vi "trace_data_compute_extra.vi"(0 "Input Trace":sgl[][](array[numeric])) -> (2 "Full Trace":sgl[][](array[numeric]))   [LabVIEW 2014]
uses:
  probe_point.ctl
  pose_source.ctl
  <vilib>/Analysis/baseanly.llb/A x Vector.vi
  initialization/micron_globals.vi
  <vilib>/Analysis/NI_AALBase.lvlib
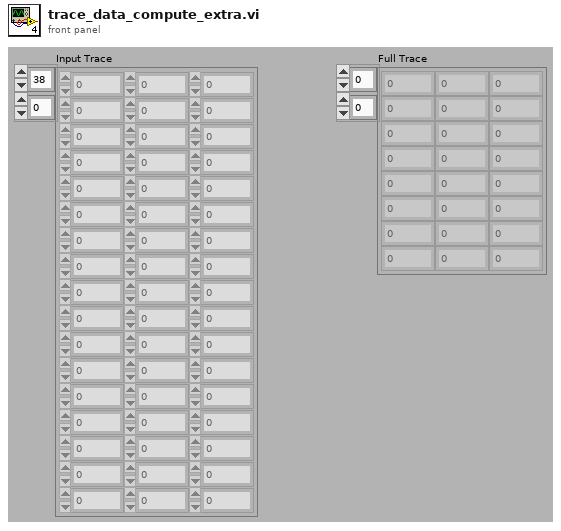
[diagram p1: front panel]
types:
  T1 = typedef "probe_point.ctl" = enum16{"Position (tip)", "Position (RCM)", "Null pos (tip)", "Null pos (RCM)", "V limiter (tip)", "V Limiter (RCM)", "Goal filter (tip)", "Goal filter (RCM)", "Goal force (tip)", "Goal force (RCM)", "Goal (tip)", "Goal (RCM)", "Link pos 0", "Link pos 1", "KF link pos 0", "KF link pos 1", "Link rate 0", "Link rate 1", "Link residue 0", "Link residue 1", "Link goal 0", "Link goal 1", "Rate limit 0", "Rate limit 1", "Link error 0", "Link error 1", "Controller 0", "Controller 1", "Output 0", "Output 1", "Drive 0", "Drive 1", "Stimulus 0", "Stimulus 1", "Trace data 0", "Trace data 1", "Analog data 0", "Analog data 1", "Status flags", "Light 0", "Light 1", "Light 2", "Light 3", "Light 4", "Light 5", "Goal origin", "Goal rotation 0", "Goal rotation 1", "Goal rotation 2", "Output origin", "Output rotation 0", "Output rotation 1", "Output rotation 2", "Handle origin", "Handle rotation 0", "Handle rotation 1", "Handle rotation 2", "Handle position", "Handle velocity", "Handle acceleration", "Handle angles", "Handle angle rates", "Handle pos residue", "Handle angle residue", "Trace length"}
  T2 = typedef "pose_source.ctl" = enum16{"Output", "Handle", "Handle KF", "Goal", "Absolute"}
  T3 = typedef "Micron params.ctl" = cluster{"Stimulus":T4, "Goal Filter A":T6, "Mode controls":T7, "Manipulator type":enum16{"Current piezo", "Voltage piezo"}, "Manipulator calibration":T8, "Network":T10, "Goal Filter B":T6, "Cancellation":T11, "Transition time":sgl, "Estimation":T13}
  T4 = typedef "stimulus.ctl" = cluster{"Type":enum16{"Off", "Step", "Sine", "Triangle", "Arbitrary"}, "Phase":dbl, "Amplitude":sgl[], "Injection point":T5, "Closed loop":bool, "Offset":sgl[], "Tip -> world":bool, "Frequency":dbl, "Length":dbl}
  T5 = typedef "injection_point.ctl" = enum16{"Total pose", "V limiter", "Goal ", "Link position", "KF link position", "Inverse kin", "Link goal", "Link error", "Controller", "Output", "Drive", "Light"}
  T6 = typedef "goal_loop_parms.ctl" = cluster{"Speedup max":sgl, "Speedup thresh":sgl, "Speedup nonlin":sgl, "Filters":cluster{"Lower Fc":sgl, "Lower Q":sgl, "Scale factor":sgl, "Upper Fc":sgl, "Upper Q":sgl, "V limit":sgl, "V limit range":sgl}[]}
  T7 = typedef "mode_conrols.ctl" = cluster{"Hold":bool, "Cancellation":bool, "Goal filter":bool, "Trigger":bool}
  T8 = typedef "manipulator_cal.ctl" = cluster{"Tool offsets":sgl[][], "Tip light calibration":T9, "Handle light calibration":T9, "Base pivots":sgl[][], "Output pivots":sgl[][], "Length center":sgl, "Workspace height":sgl[], "Workspace diameter":sgl[], "Linearization":sgl[][], "Stack travel":sgl, "Saturation pos":sgl, "Inverse filters":cluster{"filter structure":enum32{"IIR 2nd Order", "IIR 4th Order"}, "Reverse Coefficients":dbl[], "Forward Coefficients":dbl[]}[]}
  T9 = typedef "probe_calibration.ctl" = sgl[][]
  T10 = typedef "network_params.ctl" = cluster{"Remote Host":string, "Send Status":bool, "Send Port":u16, "Recv Commands":bool, "Recv Port":u16}
  T11 = typedef "sq_control_params.ctl" = cluster{"KP":T12, "KI":sgl, "KD":T12, "Max vel":sgl, "Max acc":sgl, "Int error limit":sgl, "RCM gain":sgl, "Bypass":bool, "Degraded gain":sgl}
  T12 = typedef "decoupled_gain.ctl" = cluster{"XY":sgl, "Rxy":sgl, "Z":sgl, "Rz":sgl}
  T13 = typedef "estimation_controls.ctl" = cluster{"Link":cluster{"Measure noise":dbl[], "Process noise":dbl[], "Alt process noise":dbl[], "Alt turnoff cycles":i32, "Innovation limit":dbl[], "Residue threshold":dbl, "Enable":bool}, "Handle":cluster{"Measure noise":dbl[], "Process noise":dbl[], "State limits":dbl[], "Innovation limit":dbl[], "Prediction Lookahead":sgl, "Enable":bool}}
  T14 = typedef "NI_Matrix.lvlib/RealMatrix.ctl" = dbl[][]
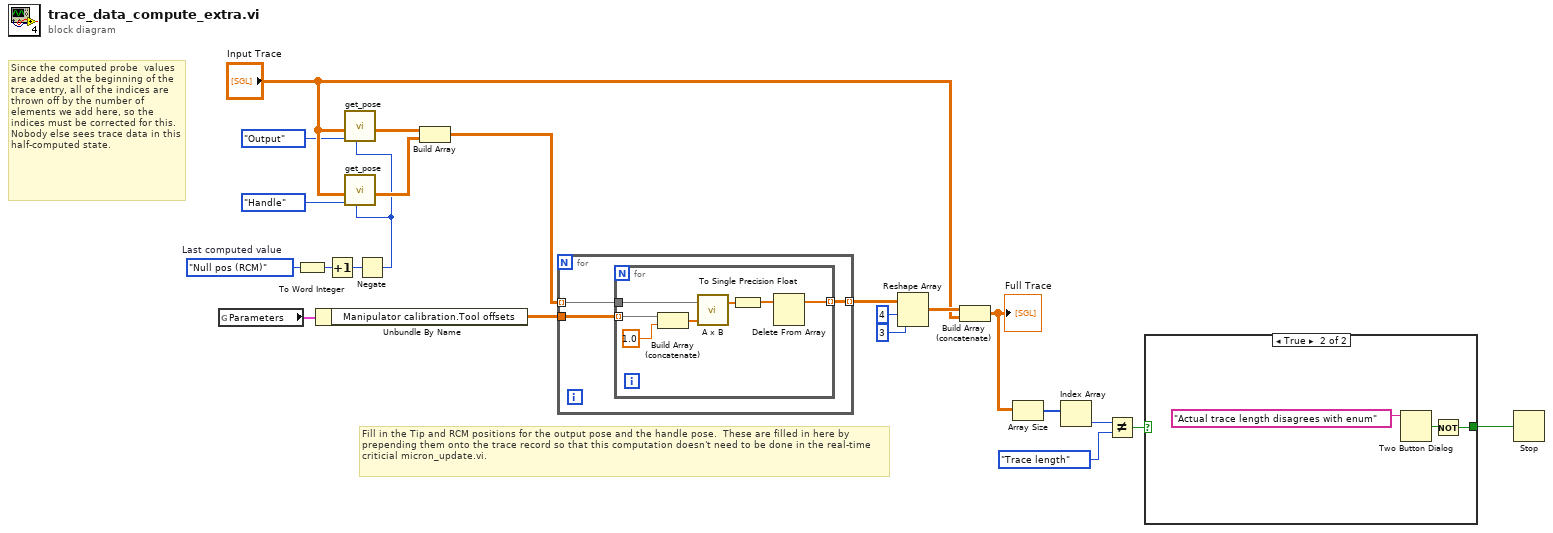
[diagram p0: block diagram]
diagram:
  w12 = probe_point."Null pos (RCM)"  # Last computed value
  # "Since the computed probe  values are added at the beginning of the trace entry, all of the indices are thrown off by the number of elements we add here, so the indices must be corrected for this.  Nobody else sees trace data in this half-computed state."
  # "Fill in the Tip and RCM positions for the output pose and the handle pose.  These are filled in here by prepending them onto the trace record so that this computation doesn't need to be done in the real-time criticial micron_update.vi."
  n1 = global read "micron_globals.vi" "Parameters"() -> (w22:T3)
  n2 = To Word Integer(number=w12) -> (16bit integer=w11:i16)
  n3 = Unbundle By Name(w22) -> ("Manipulator calibration.Tool offsets"=w13:sgl[][])
  n4 = Increment(x=w11) -> (x+1=w10:i16)
  n5 = Negate(x=w10) -> (-x=w9:i16)
  n6 = call "get_pose.vi"("Magic offset"=w9, "Selector"=pose_source."Output", "Input Trace"="Input Trace") -> ("Pose"=w21:T14)  [unwired: 8 in]
  n7 = call "get_pose.vi"("Magic offset"=w9, "Selector"=pose_source."Handle", "Input Trace"="Input Trace") -> ("Pose"=w14:T14)  [unwired: 8 in]
  n8 = Build Array(w21, w14) -> (w20:dbl[][][])
  n9 = for {
    tunnel: [w25] -> w19 mode=indexing
    tunnel: w20 -> [w23] mode=indexing
    tunnel: w13 -> [w24]
    n10 = for {
      tunnel: [w32] -> w25 mode=indexing
      tunnel: w24 -> [w27] mode=indexing
      tunnel: w23 -> [w26]
      n11 = Build Array (concatenate)(w27, sgl 1.0) -> (w30:sgl[])
      n12 = call-poly <vilib>:"A x B.vi"("Vector"=w30, "A"=w26) -> ("A x Vector"=w28:dbl[])  [unwired: 1 out]
      n13 = To Single Precision Float(number=w28) -> (single precision float=w31:sgl[])
      n14 = Delete From Array(array=w31) -> (array with subset deleted=w32:sgl[])  [unwired: 2 in, 1 out]
    }
  }
  n15 = Reshape Array(w19, 4 ("dimension size"), 3 ("dimension size")) -> (w16:sgl[][])
  n16 = Build Array (concatenate)(w16, "Input Trace") -> (w6:sgl[][])
  "Full Trace" <- w6
  n17 = Array Size(array=w6) -> (size(s)=w5:i32[])
  n18 = Index Array(array=w5) -> (element=w4:i32)  [unwired: 1 in]
  n19 = Not Equal?(x=w4, y=probe_point."Trace length") -> (x != y?=w2:bool)
  n20 = case shown="True" w2 {
    selector: w2 -> [w33 _]
    tunnel: [w33 w34] -> w1
    frame False {
    }
    frame True {
      n21 = Two Button Dialog(message="Actual trace length disagrees with enum") -> (T button?=w35:bool)  [unwired: 2 in]
      n22 = Not(x=w35) -> (.not. x?=w34:bool)
    }
  }
  n23 = Stop(stop? (T)=w1) -> ()
